vi "Second Derivative Focus Metric.vi"(7 "Image Ref (U16)":T1) -> (8 "LAP_VAR":sgl)   [LabVIEW 2016]
uses:
  <vilib>/vision/Image Controls.llb/IMAQ Image.ctl
  <vilib>/vision/NI_Vision_Development_Module.lvlib
panel:
  # "Focus metric taken from \"Diatom autofocusing in brightfield microscopy: a comparative study\" by\nJ.L. Pech-Pacheco; G. Cristobal; J. Chamorro-Martinez; J. Fernandez-Valdivia. Proceedings 15th\nInternational Conference on Pattern Recognition. ICPR-2000\n\nThis is section 3.3 Second derivative based methods."
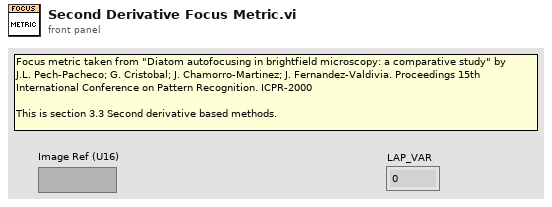
[diagram p1: front panel]
types:
  T1 = typedef "IMAQ Image.ctl" = refnum<image>
  T2 = typedef "Image Type" = u32
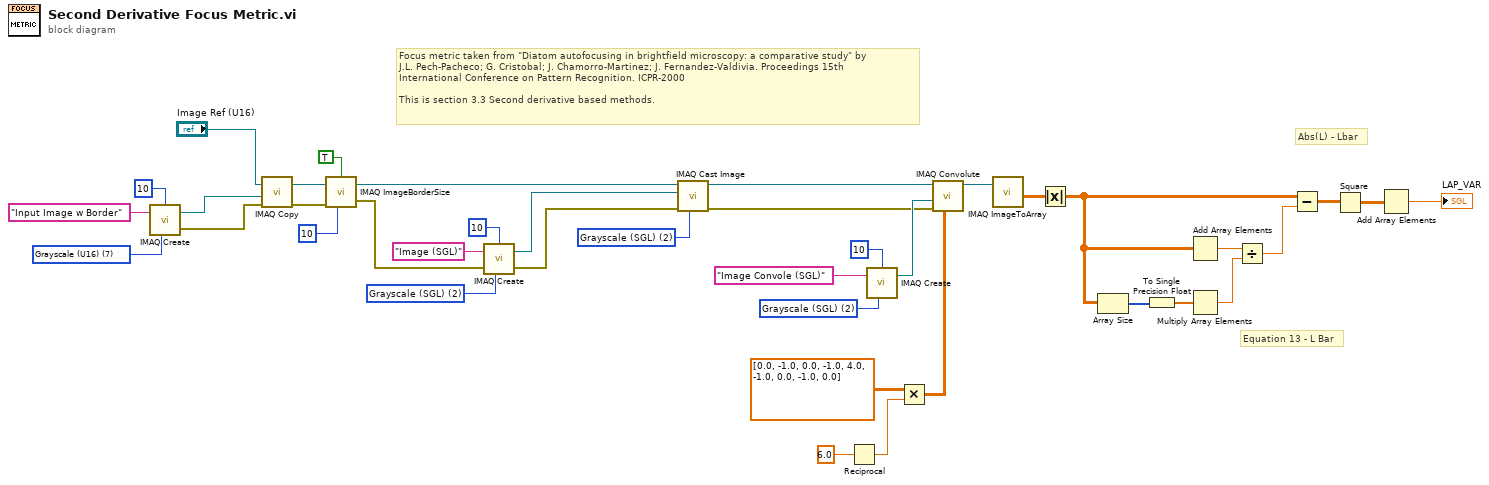
[diagram p0: block diagram]
diagram:
  w15 = T2 2 items=["Grayscale (U8)", "Grayscale (I16)", "Grayscale (SGL)", "Complex (CSG)", "RGB (U32)", "HSL (U32)", "RGB (U64)", "Grayscale (U16)"] ("Image Type")
  w22 = T2 2 items=["Grayscale (U8)", "Grayscale (I16)", "Grayscale (SGL)", "Complex (CSG)", "RGB (U32)", "HSL (U32)", "RGB (U64)", "Grayscale (U16)"] ("Image Type")
  w23 = T2 2 items=["Grayscale (U8)", "Grayscale (I16)", "Grayscale (SGL)", "Complex (CSG)", "RGB (U32)", "HSL (U32)", "RGB (U64)", "Grayscale (U16)"] ("Image Type")
  w33 = T2 7 items=["Grayscale (U8)", "Grayscale (I16)", "Grayscale (SGL)", "Complex (CSG)", "RGB (U32)", "HSL (U32)", "RGB (U64)", "Grayscale (U16)"] ("Image Type")
  # "Abs(L) - Lbar"
  # "Equation 13 - L Bar"
  # "Focus metric taken from \"Diatom autofocusing in brightfield microscopy: a comparative study\" by\nJ.L. Pech-Pacheco; G. Cristobal; J. Chamorro-Martinez; J. Fernandez-Valdivia. Proceedings 15th\nInternational Conference on Pattern Recognition. ICPR-2000\n\nThis is section 3.3 Second derivative based methods."
  n1 = call "IMAQ Create"("Border Size"=10, "Image Name"="Input Image w Border", "Image Type"=w33) -> ("New Image"=w29:T1, "error out"=w30:errorcluster)  [unwired: 2 in]
  n2 = call "IMAQ Copy"("error in (no error)"=w30, "Image Dst"=w29, "Image Src"="Image Ref (U16)") -> ("error out"=w25:errorcluster, "Image Dst Out"=w28:T1)  [unwired: 3 in]
  n3 = call "IMAQ ImageBorderSize"("Get/Set Status? (Set)"=TRUE, "Image"=w28, "Image border size in"=10, "error in (no error)"=w25) -> ("Image Out"=w17:T1, "error out"=w16:errorcluster)  [unwired: 1 out]
  n4 = call "IMAQ Create"("Border Size"=10, "Image Name"="Image (SGL)", "Image Type"=w22, "error in (no error)"=w16) -> ("New Image"=w18:T1, "error out"=w19:errorcluster)  [unwired: 1 in]
  n5 = call "IMAQ Cast Image"("Image Type"=w23, "error in (no error)"=w19, "Image Dst"=w18, "Image Src"=w17) -> ("error out"=w12:errorcluster, "Image Dst Out"=w13:T1)  [unwired: 6 in]
  n6 = Reciprocal(x=sgl 6.0) -> (1/x=w37:sgl)
  n7 = call "IMAQ Create"("Border Size"=10, "Image Name"="Image Convole (SGL)", "Image Type"=w15) -> ("New Image"=w14:T1)  [unwired: 2 in, 1 out]
  n8 = Multiply(x=sgl[][] [[0.0, -1.0, 0.0], [-1.0, 4.0, -1.0], [0.0, -1.0, 0.0]], y=w37) -> (x*y=w36:sgl[][])
  n9 = call "IMAQ Convolute"("Kernel"=w36, "error in (no error)"=w12, "Image Dst"=w14, "Image Src"=w13) -> ("Image Dst Out"=w11:T1)  [unwired: 6 in, 1 out]
  n10 = call "IMAQ ImageToArray"("Image"=w11) -> ("Image Pixels (Float)"=w3:sgl[][])  [unwired: 3 in, 4 out]
  n11 = Absolute Value(x=w3) -> (abs(x)=w2:sgl[][])
  n12 = Array Size(array=w2) -> (size(s)=w10:i32[])
  n13 = To Single Precision Float(number=w10) -> (single precision float=w9:sgl[])
  n14 = Add Array Elements(numeric array=w2) -> (sum=w8:sgl)
  n15 = Multiply Array Elements(1:w9) -> (0:w7:sgl)
  n16 = Divide(x=w8, y=w7) -> (x/y=w6:sgl)
  n17 = Subtract(x=w2, y=w6) -> (x-y=w5:sgl[][])
  n18 = Square(x=w5) -> (x^2=w4:sgl[][])
  n19 = Add Array Elements(numeric array=w4) -> (sum=→"LAP_VAR":sgl)
